vi "parseForceAndStatusResponse.vi"(8 "error in (no error)":errorcluster, 10 "DynamicFrameParser":refnum<class "DynamicFrameParser.lvclass">, 11 "DAAILC in":refnum<class "DAAILC.lvclass">) -> (0 "error out":errorcluster, 3 "DAAILC out":refnum<class "DAAILC.lvclass">)   [LabVIEW 2016, in "DAAILC.lvclass"]
uses:
  DAAILC.lvclass
  FAILC/FAILC.lvclass
  Common_RT_Modbus/DynamicFrameParser/DynamicFrameParser.lvclass
  Common_RT_Modbus/DataTypes/ExceptionCodes.ctl
  Common_RT_Modbus/RTModbus.lvlib
  D:/Code/ts_M1M3Support/Common_RT_FAILC/FAILC/FAILC.lvclass
  D:/Code/ts_M1M3Support/Common_RT_ILC/ILC/ILC.lvclass
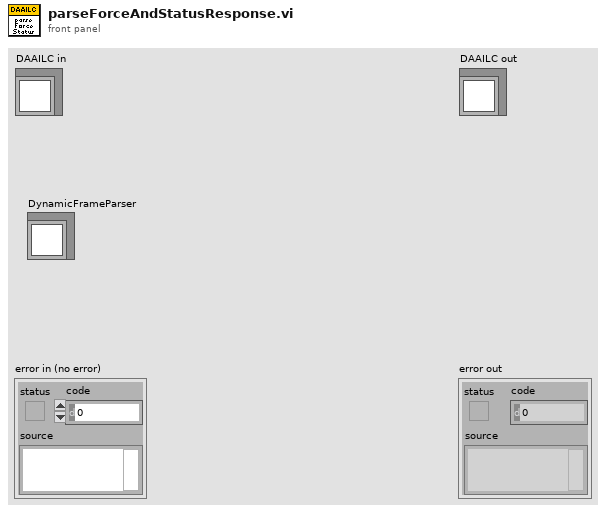
[diagram p1: front panel]
types:
  T1 = typedef "RTModbus.lvlib/ExceptionCodes.ctl" = u16
  T2 = typedef "RTFAILC.lvlib/FAData.ctl" = cluster{"Constants":T3, "Command":T5, "Telemetry":T6, "Responses":T7, "Timings":T8, "Timestamps":T9}
  T3 = typedef "RTFAILC.lvlib/FAConstants.ctl" = cluster{"ID":i16, "Type":T4}
  T4 = typedef "RTFAILC.lvlib/FATypes.ctl" = enum16{"SingleAxis", "LateralDualAxis", "CrossLateralDualAxis"}
  T5 = typedef "RTFAILC.lvlib/FACommand.ctl" = cluster{"AxialSetPoint":i32, "LateralSetPoint":i32, "AxialBoosterValveGain":sgl, "LateralBoosterValveGain":sgl}
  T6 = typedef "RTFAILC.lvlib/FATelemetry.ctl" = cluster{"ILCFault":bool, "DCAFault":bool, "BroadcastCounter":u8, "AxialLoadCellForce":sgl, "LateralLoadCellForce":sgl, "AxialBoosterValveGain":sgl, "LateralBoosterValveGain":sgl}
  T7 = typedef "RTFAILC.lvlib/FAResponses.ctl" = cluster{"BoosterValveGain":T1, "ReadBoosterValveGain":T1, "SetForce":T1, "ForceAndStatus":T1}
  T8 = typedef "RTFAILC.lvlib/FATimings.ctl" = cluster{"BroadcastSetForce":u32, "BoosterValveGain":u32, "FreezeSensorValues":u32, "ForceAndStatus":u32, "ReadBoosterValveGain":u32, "SetForce":u32}
  T9 = typedef "RTFAILC.lvlib/FATimestamps.ctl" = cluster{"BroadcastSetForce":dbl, "BoosterValveGain":dbl, "FreezeSensorValues":dbl, "ForceAndStatus":dbl, "ReadBoosterValveGain":dbl, "SetForce":dbl}
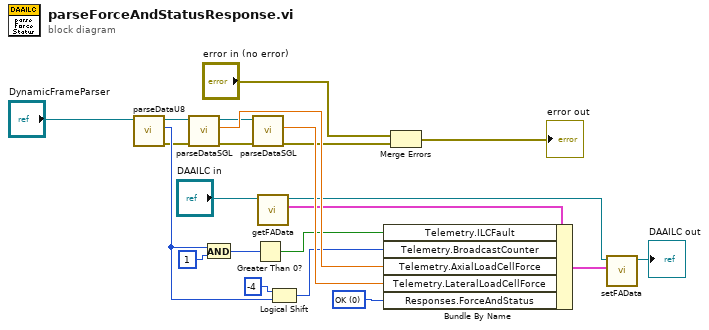
[diagram p0: block diagram]
diagram:
  w1 = T1 0 items=["OK", "IllegalFunction", "IllegalDataAddress", "IllegalDataValue", "SlaveDeviceFailure", "Acknowledge", "SlaveDeviceBusy", "NegativeAcknowledge", "MemoryParityError", "GatewayPathUnavailable", "GatewayTargetDeviceFailedToRespond"] ("FAResponses.ForceAndStatus")
  n1 = call "parseDataU8.vi"("FrameParser in"="DynamicFrameParser") -> ("error out"=w18:errorcluster, "Data"=w20:u8, "FrameParser out"=w16:refnum<class "DynamicFrameParser.lvclass">)  [unwired: 8 in]
  n2 = call "parseDataSGL.vi"("error in (no error)"=w18, "FrameParser in"=w16) -> ("error out"=w12:errorcluster, "Data"=w15:sgl, "FrameParser out"=w13:refnum<class "DynamicFrameParser.lvclass">)  [unwired: 7 in]
  n3 = And(x=w20, y=u8 1) -> (x .and. y?=w21:u8)
  n4 = call "parseDataSGL.vi"("error in (no error)"=w12, "FrameParser in"=w13) -> ("error out"=w11:errorcluster, "Data"=w14:sgl)  [unwired: 7 in, 1 out]
  n5 = Greater Than 0?(x=w21) -> (x > 0?=w3:bool)
  n6 = call "getFAData.vi"("FAILC in"="DAAILC in") -> ("FAData"=w8:T2, "FAILC out"=w6:refnum<class "DAAILC.lvclass">)  [unwired: 9 in]
  n7 = Logical Shift(y=i16 -4, x=w20) -> (x << y=w2:u8)
  n8 = Bundle By Name(cluster=w8, "Telemetry.ILCFault"=w3, "Telemetry.BroadcastCounter"=w2, "Telemetry.AxialLoadCellForce"=w15, "Telemetry.LateralLoadCellForce"=w14, "Responses.ForceAndStatus"=w1) -> (w7:T2)
  n9 = Merge Errors("error in (no error)", w11) -> (→"error out":errorcluster)
  n10 = call "setFAData.vi"("FAData"=w7, "FAILC in"=w6) -> ("FAILC out"=→"DAAILC out":refnum<class "DAAILC.lvclass">)  [unwired: 9 in]
